vi "2L17_SDEM-n0.vi"(6 "error in (no error)":errorcluster caption="errur in", 8 "N":u32, 9 "n":u32, 10 "S pop":dbl format="%.2f", 11 "s":dbl format="%.2f") -> (2 "S pop estimé":dbl, 3 "S DEM":dbl format="%.2f", 4 "error out":errorcluster caption="erreur out")   [LabVIEW 2010, in "lv_02.lvlib"]
doc: "Calcul l'écart-type de la DEM (distribution d'échantillonage des moyennes) à partir de s (écart-type de l'échantillon) ou de S (écart-type de la population) et de n (taille de l'échantillon).\nSi la population est de taille finie, câblez N\nSi l'écart type de la population est supérieur à 0, il sera choisi en priorité. Sinon, l'écart type de la population sera estimé à l'aide de l'écart type de l'achantillon"
uses:
  lv_02.lvlib
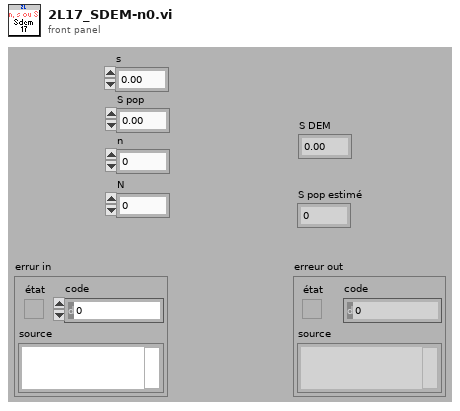
[diagram p1: front panel]
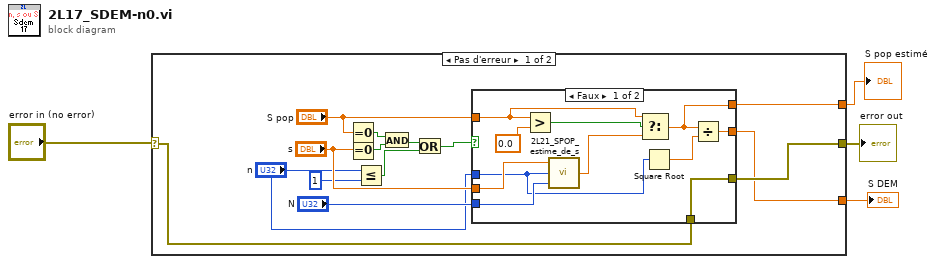
[diagram p0: block diagram]
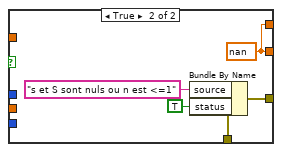
[diagram p2: hidden frame]
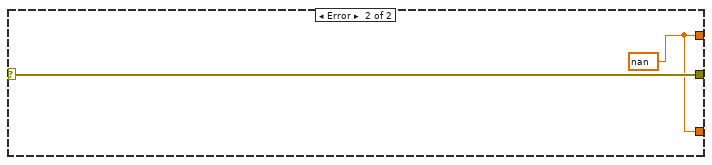
[diagram p3: hidden frame]
diagram:
  n1 = case shown="Pas d'erreur" "error in (no error)" {
    selector: "error in (no error)" -> [w9 w36]
    tunnel: [w8 w36] -> w3
    tunnel: [w6 w35] -> w2
    tunnel: [w5 w35] -> w1
    frame No Error {
      n2 = Equal To 0?(x="S pop") -> (x = 0?=w14:bool)
      n3 = Equal To 0?(x="s") -> (x = 0?=w15:bool)
      n4 = Less Or Equal?(x="n", y=u32 1) -> (x <= y?=w11:bool)
      n5 = And(x=w14, y=w15) -> (x .and. y?=w12:bool)
      n6 = Or(x=w12, y=w11) -> (x .or. y?=w10:bool)
      n7 = case shown="Faux" w10 {
        tunnel: "N" -> [w27 _]
        tunnel: [w24 w30] -> w5
        tunnel: "S pop" -> [w23 _]
        tunnel: "s" -> [w22 _]
        tunnel: "n" -> [w21 _]
        tunnel: w9 -> [w20 w34]
        tunnel: [w20 w31] -> w8
        tunnel: [w19 w30] -> w6
        frame False {
          n8 = Greater?(x=w23, y=0.0) -> (0:w28:bool)
          n9 = call "2L21_SPOP_estime_de_s.vi"("N"=w27, "n"=w21, "s"=w22) -> ("S pop estimé"=w26:dbl)
          n10 = Select(t=w23, s=w28, f=w26) -> (s? t:f=w19:dbl)
          n11 = Square Root(x=w21) -> (sqrt(x)=w25:dbl)
          n12 = Divide(x=w19, y=w25) -> (x/y=w24:dbl)
        }
        frame True {
          w30 = nan
          n13 = Bundle By Name(cluster=w34, "source"="s et S sont nuls ou n est <=1", "status"=TRUE) -> (w31:errorcluster)
        }
      }
    }
    frame Error {
      w35 = nan
    }
  }
  "error out" <- w3
  "S DEM" <- w1
  "S pop estimé" <- w2
